vi "ReadCal.vi"() -> (0 "SobrecargaC2":dbl, 2 "TermesInd":dbl[](array[numeric]) format="%#_8g", 3 "ResoExten":i8(ring) caption="Resolució Extensometre" items=["0.1", "0.2", "0.5", "0.01", "0.02", "0.05", "0.001", "0.002", "0.005"], 4 "TextTemps":string, 5 "TextDefor":string, 7 "SegonCaptador":string, 8 "TempsLectura":u16, 9 "error out":errorcluster, 10 "Idioma":string(combo), 11 "MotorBipolar":bool, 12 "UnitatsC2":string, 13 "UnitatsC1":string, 14 "Velocitat":dbl, 15 "ParoRotura":dbl, 16 "V. Retorn":dbl, 17 "PrimerCaptador":string, 18 "ViuMotor":bool, 19 "DeforActiva":bool caption="Extensòmetre Pot.", 20 "Unidades":u8(ring) items=["Kg", "N", "Lb"], 21 "Captador":u8(ring) caption="Captador utilizado:" items=["Célula 2000 Kg", "Célula Adicional"], 22 "Calibrar":bool, 23 "SobrecargaC1":dbl, 24 "Password":string, 25 "Pendents":dbl[](array[numeric]) format="%#_8g", 26 "VelocitatMàxima":dbl, 27 "PwdPrograma":string)   [LabVIEW 2017]
uses:
  <vilib>/registry/registry.llb/Registry RtKey.ctl
  <vilib>/registry/registry.llb/Read Registry Value Simple STR.vi
panel:
  out "ParoDesplazamiento":dbl
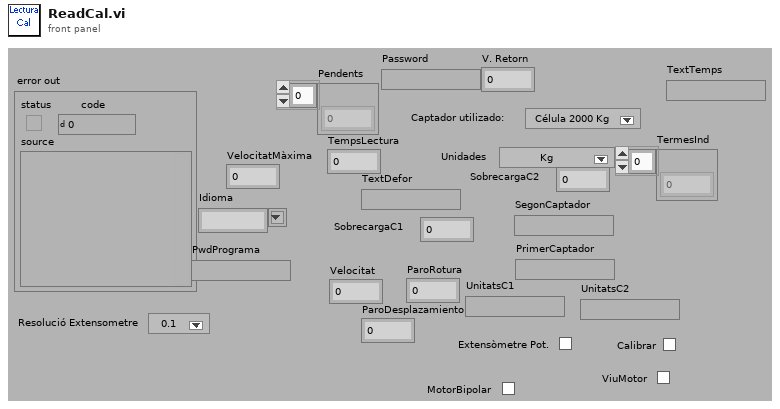
[diagram p1: front panel]
types:
  T1 = typedef "Registry RtKey.ctl" = enum32{"HKEY_CLASSES_ROOT", "HKEY_CURRENT_USER", "HKEY_LOCAL_MACHINE", "HKEY_USERS", "HKEY_PERFORMANCE_DATA", "HKEY_CURRENT_CONFIG", "HKEY_DYN_DATA"}
  T2 = typedef "Registry refnum.ctl" = refnum<k1>
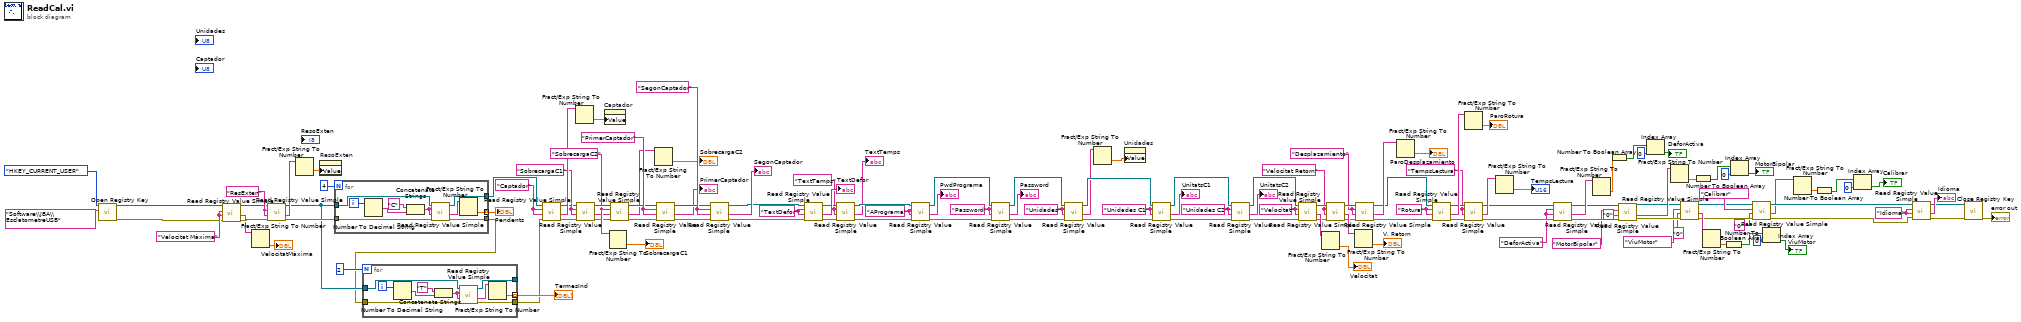
[diagram p0: block diagram]
diagram:
  w25 = "Unidades" ("value")
  w29 = "Idioma" ("value")
  w55 = "DeforActiva" ("value")
  w64 = "Velocitat Màxima" ("value")
  w67 = "ResExten" ("value")
  w69 = "TextTemps" ("value")
  w75 = "Unidades C2" ("value")
  w18 = "Desplazamiento" ("value")
  w88 = "Velocitat Retorn" ("value")
  w94 = "SobrecargaC2" ("value")
  w100 = "TextDefor" ("value")
  w105 = "TempsLectura" ("value")
  w110 = "Rotura" ("value")
  w113 = "Velocitat" ("value")
  w115 = "APrograma" ("value")
  w120 = "Password" ("value")
  w121 = "PrimerCaptador" ("value")
  w126 = "SegonCaptador" ("value")
  w131 = "SobrecargaC1" ("value")
  w132 = "Unidades C1" ("value")
  w135 = "Captador" ("value")
  n1 = call <vilib>:"Open Registry Key.vi"("subkey"="Software\\JBA\\EsclatometreUSB", "root key (HKEY_LOCAL_MACHINE)"=Registry_RtKey."HKEY_CURRENT_USER") -> ("error out"=w62:errorcluster, "refnum out"=w63:T2)  [unwired: 8 in]
  n2 = call-poly <vilib>:"Read Registry Value Simple.vi"("error in (no error)"=w62, "default data"=w64, "value"=w64, "refnum"=w63) -> ("error out"=w60:errorcluster, "String/Binary data"=w59:string, "refnum out"=w61:T2)  [unwired: 2 in, 1 out]
  n3 = Fract/Exp String To Number(string=w59) -> (number=→"VelocitatMàxima":dbl)  [unwired: 3 in, 1 out]
  n4 = call-poly <vilib>:"Read Registry Value Simple.vi"("error in (no error)"=w60, "default data"=w67, "value"=w67, "refnum"=w61) -> ("error out"=w6:errorcluster, "String/Binary data"=w66:string, "refnum out"=w5:T2)  [unwired: 2 in, 1 out]
  n5 = Fract/Exp String To Number(string=w66) -> (number=w65:dbl)  [unwired: 3 in, 1 out]
  n6 = property on="ResoExten" class="Ring (strict)"("Value"=w65) -> ()  [unwired: 2 in, 2 out]
  n7 = for {
    N: 4 -> [_]
    tunnel: w5 -> [w148]
    tunnel: w6 -> [w147]
    tunnel: [w139] -> w118 mode=indexing
    tunnel: [w143] -> w2
    tunnel: [w142] -> w136
    i -> [w146]
    n8 = Number To Decimal String(number=w146) -> (decimal integer string=w144:string)  [unwired: 1 in]
    n9 = Concatenate Strings("C" ("value"), w144) -> (w141:string)
    n10 = call-poly <vilib>:"Read Registry Value Simple.vi"("error in (no error)"=w147, "default data"=w141, "value"=w141, "refnum"=w148) -> ("error out"=w143:errorcluster, "String/Binary data"=w140:string, "refnum out"=w142:T2)  [unwired: 2 in, 1 out]
    n11 = Fract/Exp String To Number(string=w140) -> (number=w139:dbl)  [unwired: 3 in, 1 out]
  }
  "Pendents" <- w118
  n12 = for {
    N: 2 -> [_]
    tunnel: w2 -> [w158]
    tunnel: [w150] -> w3 mode=indexing
    tunnel: [w154] -> w1
    tunnel: [w153] -> _
    tunnel: w5 -> [w149]
    i -> [w157]
    n13 = Number To Decimal String(number=w157) -> (decimal integer string=w155:string)  [unwired: 1 in]
    n14 = Concatenate Strings("T" ("value"), w155) -> (w152:string)
    n15 = call-poly <vilib>:"Read Registry Value Simple.vi"("error in (no error)"=w158, "default data"=w152, "value"=w152, "refnum"=w149) -> ("error out"=w154:errorcluster, "String/Binary data"=w151:string, "refnum out"=w153:T2)  [unwired: 2 in, 1 out]
    n16 = Fract/Exp String To Number(string=w151) -> (number=w150:dbl)  [unwired: 3 in, 1 out]
  }
  "TermesInd" <- w3
  n17 = call-poly <vilib>:"Read Registry Value Simple.vi"("error in (no error)"=w1, "default data"=w135, "value"=w135, "refnum"=w136) -> ("error out"=w128:errorcluster, "String/Binary data"=w134:string, "refnum out"=w129:T2)  [unwired: 2 in, 1 out]
  n18 = Fract/Exp String To Number(string=w134) -> (number=w133:dbl)  [unwired: 3 in, 1 out]
  n19 = call-poly <vilib>:"Read Registry Value Simple.vi"("error in (no error)"=w128, "default data"=w131, "value"=w131, "refnum"=w129) -> ("error out"=w96:errorcluster, "String/Binary data"=w130:string, "refnum out"=w95:T2)  [unwired: 2 in, 1 out]
  n20 = property on="Captador" class="Ring (strict)"("Value"=w133) -> ()  [unwired: 2 in, 2 out]
  n21 = Fract/Exp String To Number(string=w130) -> (number=→"SobrecargaC1":dbl)  [unwired: 3 in, 1 out]
  n22 = call-poly <vilib>:"Read Registry Value Simple.vi"("error in (no error)"=w96, "default data"=w94, "value"=w94, "refnum"=w95) -> ("error out"=w97:errorcluster, "String/Binary data"=w93:string, "refnum out"=w98:T2)  [unwired: 2 in, 1 out]
  n23 = Fract/Exp String To Number(string=w93) -> (number=→"SobrecargaC2":dbl)  [unwired: 3 in, 1 out]
  n24 = call-poly <vilib>:"Read Registry Value Simple.vi"("error in (no error)"=w97, "default data"=w121, "value"=w121, "refnum"=w98) -> ("error out"=w123:errorcluster, "String/Binary data"=→"PrimerCaptador":string, "refnum out"=w124:T2)  [unwired: 2 in, 1 out]
  n25 = call-poly <vilib>:"Read Registry Value Simple.vi"("error in (no error)"=w123, "default data"=w126, "value"=w126, "refnum"=w124) -> ("error out"=w101:errorcluster, "String/Binary data"=→"SegonCaptador":string, "refnum out"=w102:T2)  [unwired: 2 in, 1 out]
  n26 = call-poly <vilib>:"Read Registry Value Simple.vi"("error in (no error)"=w101, "default data"=w100, "value"=w100, "refnum"=w102) -> ("error out"=w71:errorcluster, "String/Binary data"=→"TextDefor":string, "refnum out"=w70:T2)  [unwired: 2 in, 1 out]
  n27 = call-poly <vilib>:"Read Registry Value Simple.vi"("error in (no error)"=w71, "default data"=w69, "value"=w69, "refnum"=w70) -> ("error out"=w72:errorcluster, "String/Binary data"=→"TextTemps":string, "refnum out"=w73:T2)  [unwired: 2 in, 1 out]
  n28 = call-poly <vilib>:"Read Registry Value Simple.vi"("error in (no error)"=w72, "default data"=w115, "value"=w115, "refnum"=w73) -> ("error out"=w117:errorcluster, "String/Binary data"=→"PwdPrograma":string, "refnum out"=w116:T2)  [unwired: 2 in, 1 out]
  n29 = call-poly <vilib>:"Read Registry Value Simple.vi"("error in (no error)"=w117, "default data"=w120, "value"=w120, "refnum"=w116) -> ("error out"=w21:errorcluster, "String/Binary data"=→"Password":string, "refnum out"=w24:T2)  [unwired: 2 in, 1 out]
  n30 = call-poly <vilib>:"Read Registry Value Simple.vi"("error in (no error)"=w21, "default data"=w25, "value"=w25, "refnum"=w24) -> ("error out"=w22:errorcluster, "String/Binary data"=w20:string, "refnum out"=w23:T2)  [unwired: 2 in, 1 out]
  n31 = Fract/Exp String To Number(string=w20) -> (number=w19:dbl)  [unwired: 3 in, 1 out]
  n32 = property on="Unidades" class="Ring (strict)"("Value"=w19) -> ()  [unwired: 2 in, 2 out]
  n33 = call-poly <vilib>:"Read Registry Value Simple.vi"("error in (no error)"=w22, "default data"=w132, "value"=w132, "refnum"=w23) -> ("error out"=w76:errorcluster, "String/Binary data"=→"UnitatsC1":string, "refnum out"=w79:T2)  [unwired: 2 in, 1 out]
  n34 = call-poly <vilib>:"Read Registry Value Simple.vi"("error in (no error)"=w76, "default data"=w75, "value"=w75, "refnum"=w79) -> ("error out"=w77:errorcluster, "String/Binary data"=→"UnitatsC2":string, "refnum out"=w78:T2)  [unwired: 2 in, 1 out]
  n35 = call-poly <vilib>:"Read Registry Value Simple.vi"("error in (no error)"=w77, "default data"=w113, "value"=w113, "refnum"=w78) -> ("error out"=w89:errorcluster, "String/Binary data"=w111:string, "refnum out"=w90:T2)  [unwired: 2 in, 1 out]
  n36 = Fract/Exp String To Number(string=w111) -> (number=→"Velocitat":dbl)  [unwired: 3 in, 1 out]
  n37 = call-poly <vilib>:"Read Registry Value Simple.vi"("error in (no error)"=w89, "default data"=w88, "value"=w88, "refnum"=w90) -> ("error out"=w84:errorcluster, "String/Binary data"=w86:string, "refnum out"=w85:T2)  [unwired: 2 in, 1 out]
  n38 = Fract/Exp String To Number(string=w86) -> (number=→"V. Retorn":dbl)  [unwired: 3 in, 1 out]
  n39 = call-poly <vilib>:"Read Registry Value Simple.vi"("error in (no error)"=w84, "default data"=w18, "value"=w18, "refnum"=w85) -> ("error out"=w81:errorcluster, "String/Binary data"=w83:string, "refnum out"=w80:T2)  [unwired: 2 in, 1 out]
  n40 = Fract/Exp String To Number(string=w83) -> (number=→"ParoDesplazamiento":dbl)  [unwired: 3 in, 1 out]
  n41 = call-poly <vilib>:"Read Registry Value Simple.vi"("error in (no error)"=w81, "default data"=w110, "value"=w110, "refnum"=w80) -> ("error out"=w106:errorcluster, "String/Binary data"=w109:string, "refnum out"=w107:T2)  [unwired: 2 in, 1 out]
  n42 = Fract/Exp String To Number(string=w109) -> (number=→"ParoRotura":dbl)  [unwired: 3 in, 1 out]
  n43 = call-poly <vilib>:"Read Registry Value Simple.vi"("error in (no error)"=w106, "default data"=w105, "value"=w105, "refnum"=w107) -> ("error out"=w57:errorcluster, "String/Binary data"=w103:string, "refnum out"=w56:T2)  [unwired: 2 in, 1 out]
  n44 = Fract/Exp String To Number(string=w103) -> (number=→"TempsLectura":dbl)  [unwired: 3 in, 1 out]
  n45 = call-poly <vilib>:"Read Registry Value Simple.vi"("error in (no error)"=w57, "default data"=w55, "value"=w55, "refnum"=w56) -> ("error out"=w49:errorcluster, "String/Binary data"=w54:string, "refnum out"=w48:T2)  [unwired: 2 in, 1 out]
  n46 = Fract/Exp String To Number(string=w54) -> (number=w53:dbl)  [unwired: 3 in, 1 out]
  n47 = Number To Boolean Array(number=w53) -> (Boolean array=w52:bool[])
  n48 = call-poly <vilib>:"Read Registry Value Simple.vi"("error in (no error)"=w49, "default data"="0", "value"="MotorBipolar", "refnum"=w48) -> ("error out"=w40:errorcluster, "String/Binary data"=w44:string, "refnum out"=w41:T2)  [unwired: 2 in, 1 out]
  n49 = Index Array(array=w52, index=0) -> (element=→"DeforActiva":bool)
  n50 = Fract/Exp String To Number(string=w44) -> (number=w47:dbl)  [unwired: 3 in, 1 out]
  n51 = call-poly <vilib>:"Read Registry Value Simple.vi"("error in (no error)"=w40, "default data"="0", "value"="ViuMotor", "refnum"=w41) -> ("error out"=w16:errorcluster, "String/Binary data"=w38:string, "refnum out"=w13:T2)  [unwired: 2 in, 1 out]
  n52 = Number To Boolean Array(number=w47) -> (Boolean array=w46:bool[])
  n53 = Fract/Exp String To Number(string=w38) -> (number=w34:dbl)  [unwired: 3 in, 1 out]
  n54 = Number To Boolean Array(number=w34) -> (Boolean array=w37:bool[])
  n55 = Index Array(array=w46, index=0) -> (element=→"MotorBipolar":bool)
  n56 = call-poly <vilib>:"Read Registry Value Simple.vi"("error in (no error)"=w16, "default data"="0", "value"="Calibrar", "refnum"=w13) -> ("error out"=w17:errorcluster, "String/Binary data"=w9:string, "refnum out"=w12:T2)  [unwired: 2 in, 1 out]
  n57 = Index Array(array=w37, index=0) -> (element=→"ViuMotor":bool)
  n58 = Fract/Exp String To Number(string=w9) -> (number=w10:dbl)  [unwired: 3 in, 1 out]
  n59 = Number To Boolean Array(number=w10) -> (Boolean array=w8:bool[])
  n60 = Index Array(array=w8, index=0) -> (element=→"Calibrar":bool)
  n61 = call-poly <vilib>:"Read Registry Value Simple.vi"("error in (no error)"=w17, "default data"=w29, "value"=w29, "refnum"=w12) -> ("error out"=w26:errorcluster, "String/Binary data"=→"Idioma":string, "refnum out"=w27:T2)  [unwired: 2 in, 1 out]
  n62 = call <vilib>:"Close Registry Key.vi"("error in (no error)"=w26, "refnum"=w27) -> ("error out"=→"error out":errorcluster)  [unwired: 5 in]
